vi "POP Read to DOT-CRLF.vi"(3 "error in":errorcluster, 5 "connection ID in":refnum<k5>) -> (0 "error out":errorcluster, 1 "LIST response":string="\r\n", 2 "connection ID out":refnum<k5>)   [LabVIEW 2012]
doc: "This is a POP utility VI designed to continue reading characters from a mail server via TCP/IP until it reads the following sequence of characters: period (.), carriage-return, linefeed.\n\nThis sequence is the termination code from a POP mail server to indicate that the end of a mail file has been reached."
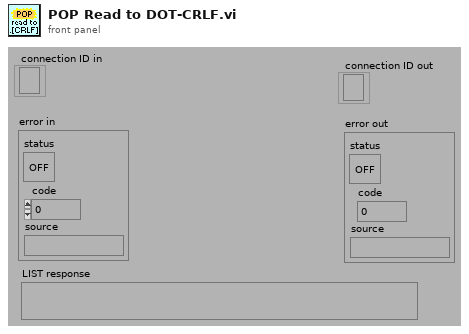
[diagram p1: front panel]
types:
  T1 = enum16{"Standard", "Buffered", "CRLF", "Immediate"}
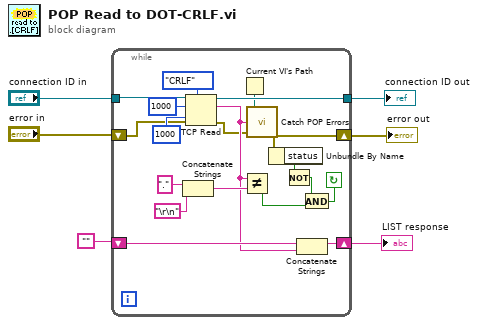
[diagram p0: block diagram]
diagram:
  n1 = while {
    tunnel: [w15] -> w1
    shift-left: "error in" -> [w21]
    shift-right: [w10] -> w3
    tunnel: "connection ID in" -> [w22]
    shift-left: "" -> [w17]
    shift-right: [w16] -> w2
    stop <- w14 continue-if-true
    n2 = Concatenate Strings(".", "\r\n") -> (w18:string)
    n3 = TCP Read(connection ID=w22, bytes to read=1000, error in (no error)=w21, 7:T1."CRLF" ("mode (standard)"), 9:1000 ("timeout ms (25000)")) -> (connection ID out=w15:refnum<k5>, data out=w12:string, error out=w11:errorcluster)
    n4 = Current VI's Path() -> (path=w13:path)
    n5 = Not Equal?(x=w12, y=w18) -> (x != y?=w8:bool)
    n6 = call "Catch POP Errors.vi"("error in"=w11, "POP server response"=w12, "Caller Path"=w13) -> ("error out"=w10:errorcluster)
    n7 = Unbundle By Name(w10) -> ("status"=w9:bool)
    n8 = Not(x=w9) -> (.not. x?=w7:bool)
    n9 = Concatenate Strings(w17, w12) -> (w16:string)
    n10 = And(x=w7, y=w8) -> (x .and. y?=w14:bool)
  }
  "error out" <- w3
  "LIST response" <- w2
  "connection ID out" <- w1
